vi "step rk4.vi"(4 "F initial":dbl[](array[numeric]), 5 "dt":dbl=1.0, 6 "y initial":dbl[](array[numeric]), 7 "reset":bool, 8 "error in (no error)":errorcluster, 9 "params":dbl[](array[numeric]), 10 "time dependent fcn":dbl[](array[numeric]), 11 "ODE fcn ref":refnum<vi>) -> (0 "error out":errorcluster, 3 "y out":dbl[](array[numeric]))   [LabVIEW 2012, in "common.lvlib"]
uses:
  common.lvlib
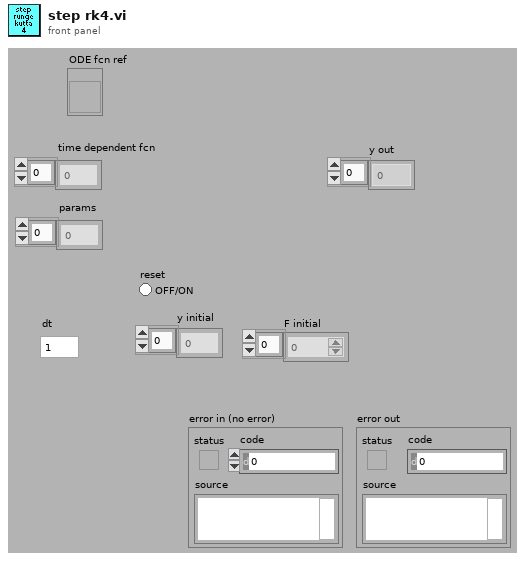
[diagram p1: front panel]
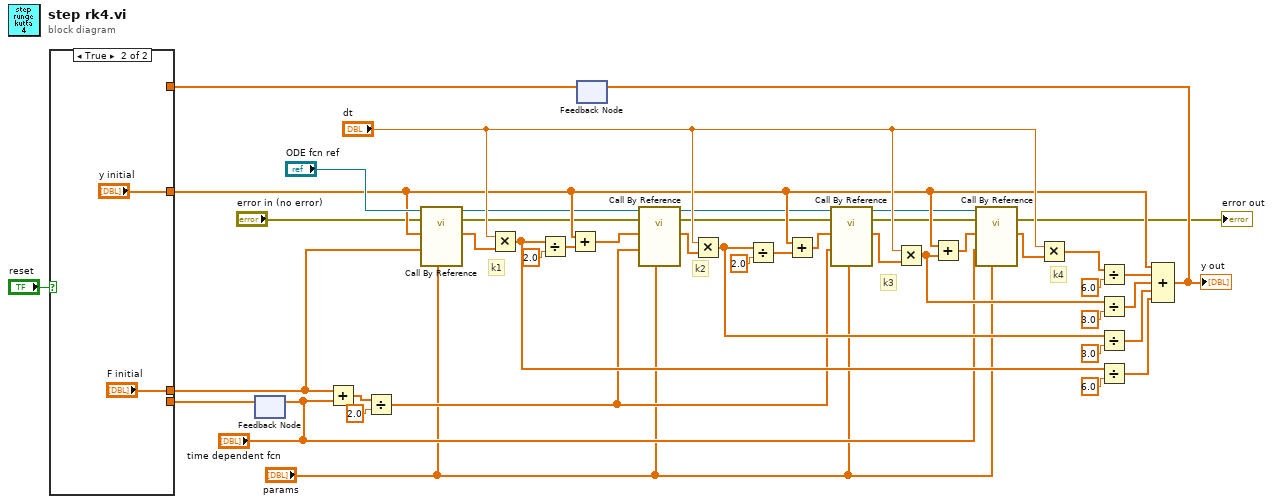
[diagram p0: block diagram]
diagram:
  # "k4"
  # "k3"
  # "k2"
  # "k1"
  n1 = feedback-in #1("time dependent fcn") -> ()
  n2 = feedback #1() -> (w22:dbl[])  [unwired: 1 in]
  n3 = feedback #2() -> (w23:dbl[])  [unwired: 1 in]
  n4 = case shown="True" "reset" {
    tunnel: [w46 "y initial"] -> w20
    tunnel: [w45 "F initial"] -> w19
    tunnel: w23 -> [w46 _]
    tunnel: w22 -> [w45 _]
    frame False {
    }
    frame True {
    }
  }
  n5 = Add(x=w19, y="time dependent fcn") -> (x+y=w43:dbl[])
  n6 = Divide(x=w43, y=2.0) -> (x/y=w11:dbl[])
  n7 = call-by-ref "?"(reference="ODE fcn ref", error in="error in (no error)", "params"="params", "F"=w19, "y"=w20) -> (reference out=w16:refnum<vi>, error out=w15:errorcluster, "dydt"=w17:dbl[])  [unwired: 8 in]
  n8 = Multiply(x="dt", y=w17) -> (x*y=w33:dbl[])
  n9 = Divide(x=w33, y=2.0) -> (x/y=w34:dbl[])
  n10 = Add(x=w20, y=w34) -> (x+y=w14:dbl[])
  n11 = call-by-ref "?"(reference=w16, error in=w15, "params"="params", "F"=w11, "y"=w14) -> (reference out=w4:refnum<vi>, error out=w3:errorcluster, "dydt"=w13:dbl[])  [unwired: 8 in]
  n12 = Multiply(x="dt", y=w13) -> (x*y=w31:dbl[])
  n13 = Divide(x=w31, y=2.0) -> (x/y=w30:dbl[])
  n14 = Add(x=w20, y=w30) -> (x+y=w12:dbl[])
  n15 = call-by-ref "?"(reference=w4, error in=w3, "params"="params", "F"=w11, "y"=w12) -> (reference out=w5:refnum<vi>, error out=w2:errorcluster, "dydt"=w10:dbl[])  [unwired: 8 in]
  n16 = Multiply(x="dt", y=w10) -> (x*y=w39:dbl[])
  n17 = Add(x=w20, y=w39) -> (x+y=w9:dbl[])
  n18 = call-by-ref "?"(reference=w5, error in=w2, "params"="params", "F"="time dependent fcn", "y"=w9) -> (error out=→"error out":errorcluster, "dydt"=w6:dbl[])  [unwired: 8 in, 1 out]
  n19 = Multiply(x="dt", y=w6) -> (x*y=w37:dbl[])
  n20 = Divide(x=w37, y=6.0) -> (x/y=w29:dbl[])
  n21 = Divide(x=w39, y=3.0) -> (x/y=w28:dbl[])
  n22 = Divide(x=w31, y=3.0) -> (x/y=w27:dbl[])
  n23 = Divide(x=w33, y=6.0) -> (x/y=w26:dbl[])
  n24 = Compound Arithmetic op=ADD(w20, w29, w28, w27, w26) -> (w24:dbl[])
  "y out" <- w24
  n25 = feedback-in #2(w24) -> ()
